vi "MouseDown Response.vi"(4 "PlatMods":T1, 6 "Mods":cluster{"Double Click":bool, "Menu Key":bool}, 8 "error in (no error)":errorcluster, 9 "Button":u16, 10 "Coords":T2, 11 "Editor Handler in":refnum<class "Imager Handler.lvclass">) -> (0 "error out":errorcluster, 3 "Editor Handler out":refnum<class "Imager Handler.lvclass">)   [LabVIEW 2016, in "Imager Handler.lvclass"]
uses:
  Imager Handler.lvclass
  C:/Program Files (x86)/National Instruments/LabVIEW 2016/vi.lib/LIEF/Image Editor Handler/Image Editor Handler.lvclass
  <vilib>/Utility/miscctls.llb/LVPoint32TypeDef.ctl
  <vilib>/LIEF/Image Editor Handler/Image Editor Handler.lvclass/Image Editor Handler.ctl
  Imager Handler.lvclass/Imager Handler.ctl
  <vilib>/LIEF/Image Editor Handler/Read PictureRef.vi
  <vilib>/LIEF/Image Editor Handler/Read Shapes.vi
  <vilib>/LIEF/Image Editor Handler/Image Editor Handler.lvclass
  <vilib>/LIEF/Forms/Shape/Shape.lvclass
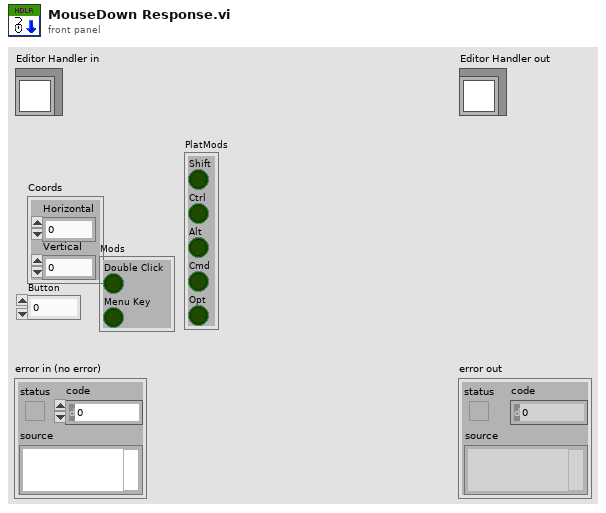
[diagram p1: front panel]
types:
  T1 = cluster{"Shift":bool, "Ctrl":bool, "Alt":bool, "Cmd":bool, "Opt":bool}
  T2 = typedef "LVPoint32TypeDef.ctl" = cluster{"Horizontal":i32, "Vertical":i32}
  T3 = typedef "LVPositionTypeDef.ctl" = cluster{"Left":i32, "Top":i32}
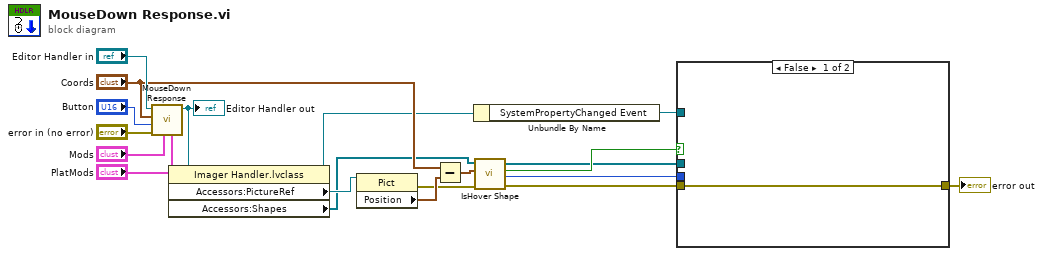
[diagram p0: block diagram]
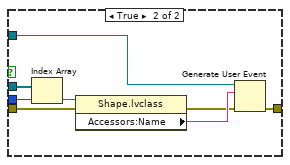
[diagram p2: hidden frame]
diagram:
  n1 = call-parent "MouseDown Response.vi"("PlatMods"="PlatMods", "Mods"="Mods", "error in (no error)"="error in (no error)", "Button"="Button", "Coords"="Coords", "Editor Handler in"="Editor Handler in") -> ("Editor Handler out"=w10:refnum<class "Imager Handler.lvclass">)  [unwired: 4 in, 1 out]
  "Editor Handler out" <- w10
  n2 = property class="Imager Handler.lvclass"(reference=w10) -> (reference out=w7:refnum<class "Imager Handler.lvclass">, "Accessors:PictureRef"=w9:refnum<vi>, "Accessors:Shapes"=w8:refnum<data-value>[])  [unwired: 1 in, 1 out]
  n3 = property class="Pict"(reference=w9) -> (error out=w12:errorcluster, "Position"=w14:T3)  [unwired: 1 in, 1 out]
  n4 = Subtract(x="Coords", y=w14) -> (x-y=w13:T2)
  n5 = Unbundle By Name(w7) -> ("SystemPropertyChanged Event"=w3:refnum<user-event>)
  n6 = call <vilib>:"IsHover Shape.vi"("error in (no error)"=w12, "Coords"=w13, "Shape in"=w8) -> ("error out"=w2:errorcluster, "Node ID"=w4:i32, "Found?"=w6:bool, "Shape out"=w5:refnum<data-value>[])  [unwired: 3 in, 2 out]
  n7 = case shown="False" w6 {
    tunnel: w5 -> [_ w28]
    tunnel: w4 -> [_ w27]
    tunnel: w3 -> [_ w25]
    tunnel: w2 -> [w20 w22]
    tunnel: [w20 w21] -> w1
    frame False {
    }
    frame True {
      n8 = Index Array(array=w28, index=w27) -> (element=w26:refnum<data-value>)
      n9 = property class="Shape.lvclass"(reference=w26, error in=w22) -> (error out=w23:errorcluster, "Accessors:Name"=w24:string)  [unwired: 1 out]
      n10 = Generate User Event(user event=w25, event data cluster=w24, error in=w23) -> (error out=w21:errorcluster)  [unwired: 1 in, 1 out]
    }
  }
  "error out" <- w1
